vi "Test - Template.vi"   [LabVIEW 2020, in "JSON Schema Generator.lvlib"]
uses:
  JSON Schema Generator.lvlib
  <vilib>/addons/_JKI Toolkits/Caraya/classes/Test/Test.lvclass
  <vilib>/addons/_JKI Toolkits/Caraya/classes/Assert/Assert.lvclass
  <vilib>/addons/_JKI Toolkits/Caraya/classes/Assert/Assert Not Error.vi
  <vilib>/addons/_JKI Toolkits/Caraya/classes/Assert/Assert True.vi
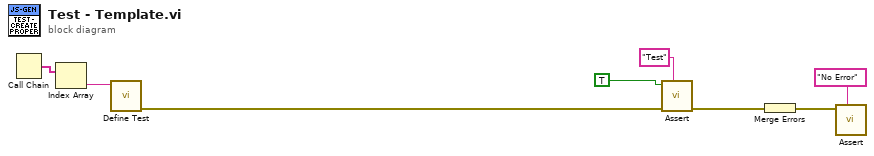
[diagram p0: block diagram]
diagram:
  n1 = Call Chain() -> (call chain=w8:string[])
  n2 = Index Array(array=w8) -> (element=w7:string)  [unwired: 1 in]
  n3 = call <vilib>:"Define Test.vi"("Label (VI Title)"=w7) -> ("error out"=w1:errorcluster)  [unwired: 9 in, 1 out]
  n4 = call-poly <vilib>:"Assert.vi"("Label"="Test", "error in (no error)"=w1, "True?"=TRUE) -> ("error out"=w5:errorcluster)  [unwired: 7 in, 1 out]
  n5 = Merge Errors(w5) -> (w3:errorcluster)
  n6 = call-poly <vilib>:"Assert.vi"("Label"="No Error", "Not Error?"=w3) -> ()  [unwired: 8 in, 2 out]
